vi "Current Directory.vi"(10 "error in (no error)":errorcluster) -> (2 "error out":errorcluster, 3 "Current Directory":path)   [LabVIEW 2020, in "neg-pkg-cli.lvlib" / "CLI.lvclass"]
uses:
  CLI.lvclass
  kernel32.dll
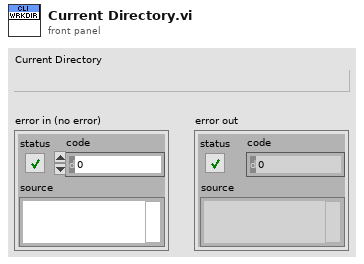
[diagram p1: front panel]
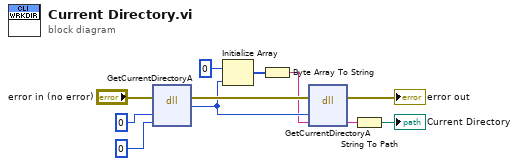
[diagram p0: block diagram]
diagram:
  n1 = dll-call lib="kernel32.dll" fn="GetCurrentDirectoryA" label="GetCurrentDirectory"(error in="error in (no error)", "nBufferLength"=0, "lpBuffer"=u32 0) -> (error out=w11:errorcluster, "return type"=w7:i32)  [unwired: 4 in, 1 out]
  n2 = Initialize Array(u8 0 ("element"), w7) -> (w9:u8[])
  n3 = Byte Array To String(unsigned byte array=w9) -> (string=w6:string)
  n4 = dll-call lib="kernel32.dll" fn="GetCurrentDirectoryA" label="GetCurrentDirectory"(error in=w11, "nBufferLength"=w7, "Directory"=w6) -> (error out=→"error out":errorcluster, "Directory"=w8:string)  [unwired: 4 in, 1 out]
  n5 = String To Path(string=w8) -> (path=→"Current Directory":path)
